vi "NG_CONTENT.vi"() -> (0 "STR 2":string caption="STR")   [LabVIEW 2017]
panel:
  in  "STR":string
  # "NG CONTENT:"
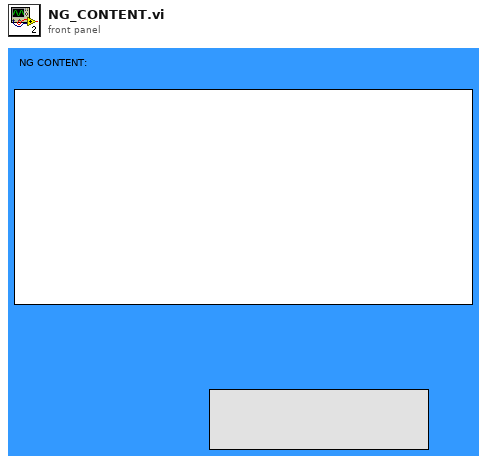
[diagram p1: front panel]
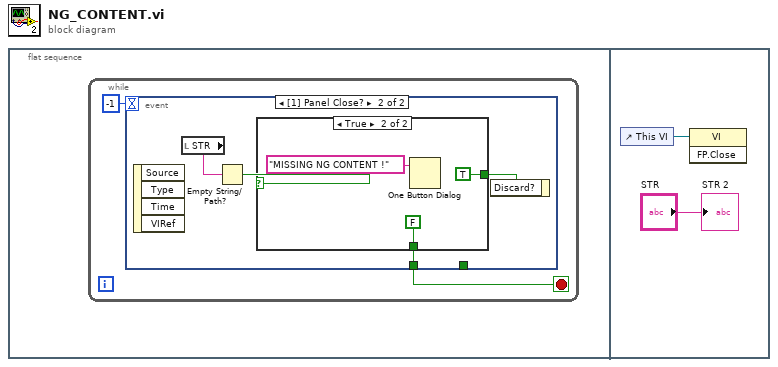
[diagram p0: block diagram]
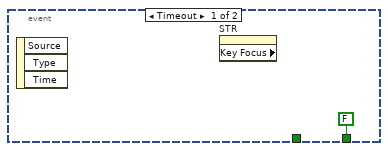
[diagram p2: hidden frame]
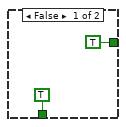
[diagram p3: hidden frame]
diagram:
  n1 = flat-sequence {
    frame #0 {
      n2 = while {
        stop <- w1 stop-if-true
        n3 = event shown="[1] Panel Close?" {
          selector: _ -> [_ _]
          dyn-events: _ -> [_ _]
          timeout: -1 -> [_ _]
          tunnel: [FALSE _] -> _
          tunnel: [_ w5] -> w1
          event Timeout {
            n4 = event-data() -> ()  [unwired: 1 in, 3 out]
            n5 = property on="STR" class="Str" props=["Key Focus"]() -> ()  [unwired: 2 in, 3 out]
          }
          event Panel Close? {
            n6 = event-data() -> ()  [unwired: 1 in, 4 out]
            n7 = local read "STR"() -> (w7:string)
            n8 = Empty String/Path?(string/path=w7) -> (empty?=w6:bool)
            n9 = case shown="True" w6 {
              tunnel: [TRUE FALSE] -> w5
              tunnel: [TRUE ("Discard?") TRUE ("Discard?")] -> w4
              frame False {
              }
              frame True {
                n10 = One Button Dialog(message="MISSING NG CONTENT !") -> ()  [unwired: 1 in, 1 out]
              }
            }
            n11 = event-data("Discard?"=w4) -> ()  [unwired: 1 in, 1 out]
          }
        }
      }
    }
    frame #1 {
      n12 = control-ref of="This VI"() -> (w14:refnum<vi>)
      n13 = invoke class="VI" method="FP.Close"(reference=w14) -> ()  [unwired: 2 in, 3 out]
      "STR 2" <- "STR"
    }
  }
